vi "CANOpen_Main_Emergency.vi"(6 "EM GB NG conf":T3(array[cluster])=[{"Emergency"={"Enable"=TRUE}, "Heartbeat and Node Guarding"={"Mode"=enum."None", "Guard Time (ms)"=5, "Consumer Time (ms)"=5}}, {"Emergency"={"Enable"=TRUE}, "Heartbeat and Node Guarding"={"Mode"=enum."None", "Guard Time (ms)"=5, "Consumer Time (ms)"=5}}], 7 "Period":i64=10, 8 "error in (no error)":errorcluster, 9 "stop in":bool, 10 "Nodes":T4[](array[typedef])=[{"RPDOs"=[], "TPDOs"=[], "Node ID"=1, "SDOs"=[], "Dynamic SDOs"=[], "Node run state"=128, "Emergency"=FALSE, "HB NG"={"Mode"=enum."None", "Update Time"=5, "Static detect in None"=enum."HB"}, "Delay for opp. state (ms)"=1000.0, "Node init static SDO state"=128, "Stop and Reset on Shutdown"=FALSE}, {"RPDOs"=[], "TPDOs"=[], "Node ID"=2, "SDOs"=[], "Dynamic SDOs"=[], "Node run state"=128, "Emergency"=FALSE, "HB NG"={"Mode"=enum."None", "Update Time"=5, "Static detect in None"=enum."HB"}, "Delay for opp. state (ms)"=1000.0, "Node init static SDO state"=128, "Stop and Reset on Shutdown"=FALSE}] {"Node init static SDO state" items=["start remote node"=1, "enter pre-operational"=128]; "Node run state" items=["start remote node"=1, "stop remote node"=2, "enter pre-operational"=128, "reset node"=129, "reset communication"=130]; "RPDOs"."PDO Channel" items=["PDO 1", "PDO 2", "PDO 3", "PDO 4"]; "RPDOs"."Parameters"."Bit Offset" max=8 step=1; "RPDOs"."Parameters"."Byte Offset" max=8 step=1; "TPDOs"."PDO Channel" items=["PDO 1", "PDO 2", "PDO 3", "PDO 4"]; "TPDOs"."Parameters"."Bit Offset" max=8 step=1; "TPDOs"."Parameters"."Byte Offset" max=8 step=1}, 11 "interface object in":refnum<k20>) -> (0 "error out":errorcluster, 1 "Timestamp":timestamp, 2 "emergency message":T11 {"manufacturer specific error field" format="%.0x"; "error register" format="%.0x"; "error code" format="%.0x"}, 3 "interface object out":refnum<k20>, 5 "Is New?":bool)   [LabVIEW 2013, in "CANOpen Addon Custom Device.lvlib"]
uses:
  CANOpen Addon Custom Device.lvlib
  SubVIS/CANOpen_Node Message Settings.ctl
  Shared Code/CANOpen_PDO Settings.ctl
  Shared Code/CANOpen_PDO Parameter Settings.ctl
  Shared Code/CANOpen_PDO Data Type.ctl
  Shared Code/CANOpen_SDO Settings.ctl
  CanOpen_NMT_Config.ctl
  CanOpen_NMT_Static detect.ctl
  Shared Code/CANOpen_Emergency Settings.ctl
  Shared Code/CANOpen_Heartbeat and Node Guarding Settings.ctl
  Emergency VI states.ctl
  <vilib>/Platform/TimedLoop/XDataNode/timing_clust.ctl
  <vilib>/Platform/TimedLoop/XDataNode/nitl_modes.ctl
  <vilib>/Platform/TimedLoop/XDataNode/wakeup.ctl
  <vilib>/CANopenLib/CANOPEN.llb/CANopen Heartbeat Create.vi
  <vilib>/CANopenLib/CANOPEN.llb/CANopen Heartbeat Start.vi
  <vilib>/CANopenLib/CANOPEN.llb/CANopen Heartbeat State Read.vi
  <vilib>/CANopenLib/CANOPEN.llb/CANopen Heartbeat Close.vi
  <vilib>/CANopenLib/CANOPEN.llb/CANopen Emergency Create.vi
  <vilib>/CANopenLib/CANOPEN.llb/CANopen Emergency Start.vi
  <vilib>/CANopenLib/CANOPEN.llb/CANopen Emergency Read.vi
  <vilib>/CANopenLib/CANOPEN.llb/CANopen Emergency Close.vi
  <vilib>/CANopenLib/CANOPEN.llb/CANopen Node Guarding Create.vi
  <vilib>/CANopenLib/CANOPEN.llb/CANopen Node Guarding Start.vi
  <vilib>/CANopenLib/CANOPEN.llb/CANopen Node Guarding State Read.vi
  <vilib>/CANopenLib/CANOPEN.llb/CANopen Node Guarding Close.vi
  <vilib>/Platform/TimedLoop/XDataNode/XDataNode.xnode
  <vilib>/Platform/TimedLoop/XDataNode/XDNodeRunTimeDep.lvlib
panel:
  out "timestamp 2":timestamp
  out "state 2":u16(ring) items=["unknown"=1, "bootup"=0, "stopped"=4, "operational"=5, "pre-operational"=127, "connection lost"=128]
  out "error out 3":errorcluster
  out "state":u16(ring) items=["unknown"=1, "bootup"=0, "stopped"=4, "operational"=5, "pre-operational"=127, "connection lost"=128]
  out "timestamp":timestamp
  out "error out 2":errorcluster
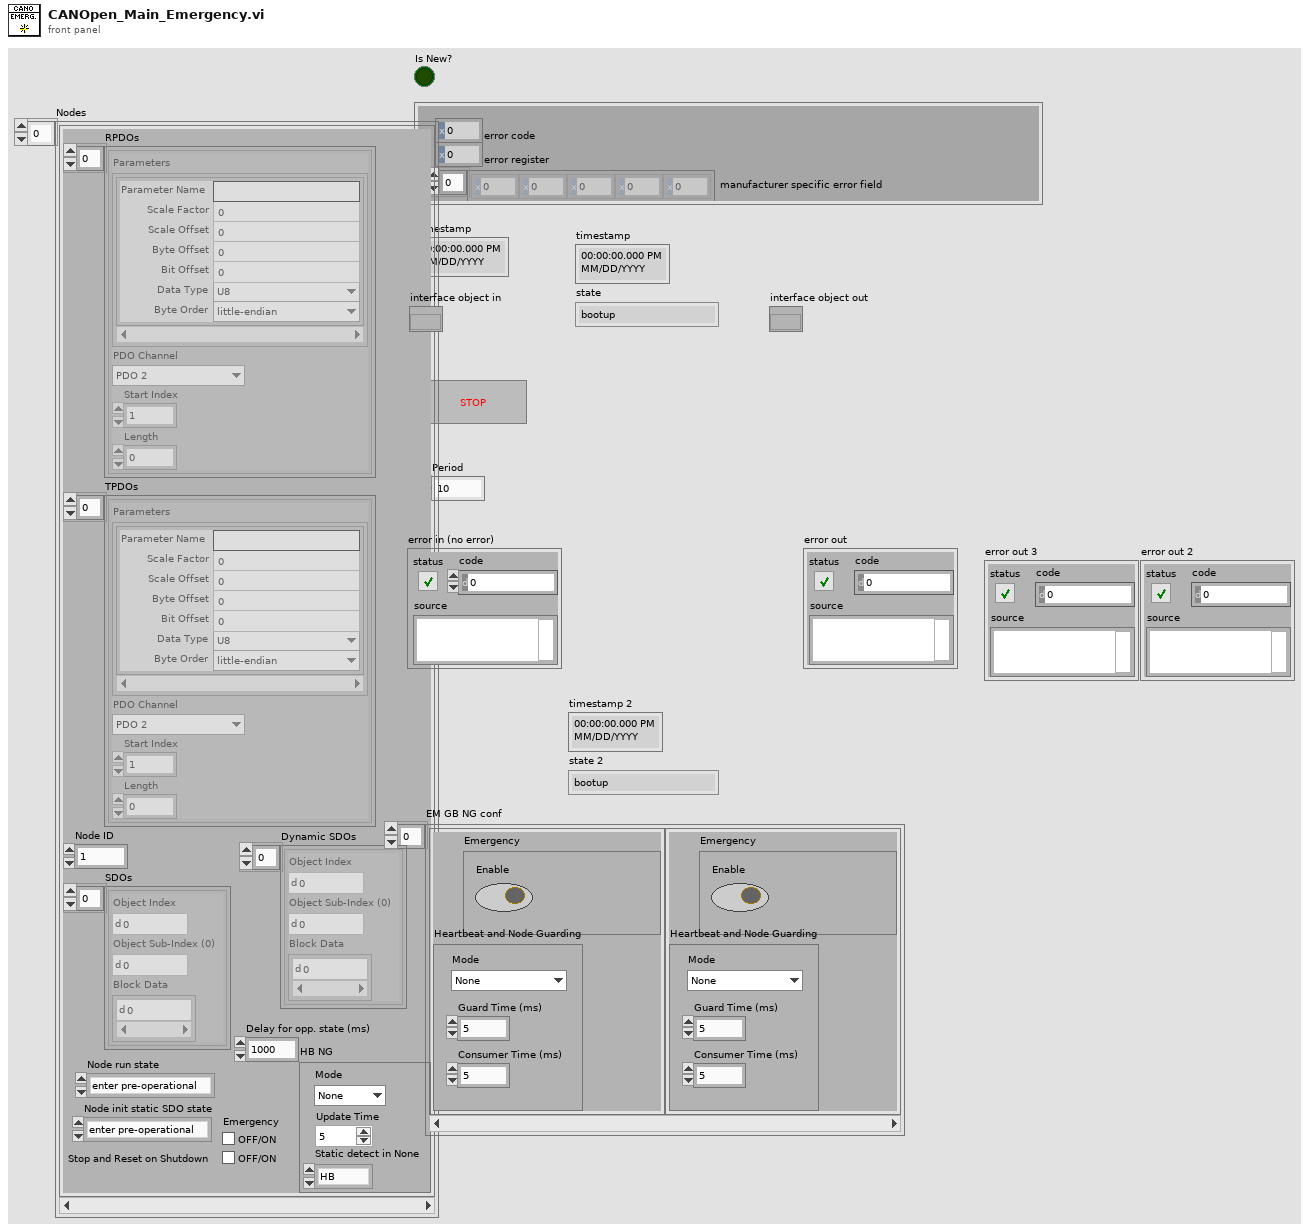
[diagram p1: front panel]
types:
  T1 = typedef "CANOpen Addon Custom Device.lvlib/CANOpen_Emergency Settings.ctl" = cluster{"Enable":bool}
  T2 = typedef "CANOpen Addon Custom Device.lvlib/CANOpen_Heartbeat and Node Guarding Settings.ctl" = cluster{"Mode":enum16{"None", "Hearbeat", "Node Guarding"}, "Guard Time (ms)":u16, "Consumer Time (ms)":u16}
  T3 = cluster{"Emergency":T1, "Heartbeat and Node Guarding":T2}[]
  T4 = typedef "CANOpen_Node Message Settings.ctl" = cluster{"RPDOs":T5[], "TPDOs":T5[], "Node ID":u8, "SDOs":T8[], "Dynamic SDOs":T8[], "Node run state":u16, "Emergency":bool, "HB NG":T9, "Delay for opp. state (ms)":dbl, "Node init static SDO state":u16, "Stop and Reset on Shutdown":bool}
  T5 = typedef "CANOpen Addon Custom Device.lvlib/CANOpen_PDO Settings.ctl" = cluster{"Parameters":T6[], "PDO Channel":u8, "Start Index":u32, "Length":u32}
  T6 = typedef "CANOpen Addon Custom Device.lvlib/CANOpen_PDO Parameter Settings.ctl" = cluster{"Parameter Name":string, "Scale Factor":dbl, "Scale Offset":dbl, "Byte Offset":u8, "Bit Offset":u8, "Data Type":T7, "Byte Order":enum16{"big-endian, network order", "little-endian"}}
  T7 = typedef "CANOpen Addon Custom Device.lvlib/CANOpen_PDO Data Type.ctl" = enum16{"U8", "U16", "U32", "I8", "I16", "I32", "Single", "Double", "Boolean"}
  T8 = typedef "CANOpen Addon Custom Device.lvlib/CANOpen_SDO Settings.ctl" = cluster{"Object Index":u16, "Object Sub-Index (0)":u8, "Block Data":u8[]}
  T9 = typedef "CANOpen Addon Custom Device.lvlib/CanOpen_NMT_Config.ctl" = cluster{"Mode":enum16{"None", "HB", "NG"}, "Update Time":u16, "Static detect in None":T10}
  T10 = typedef "CANOpen Addon Custom Device.lvlib/CanOpen_NMT_Static detect.ctl" = enum16{"None", "HB", "NG"}
  T11 = cluster{"error code":u16, "error register":u8, "manufacturer specific error field":u8[]}
  T12 = typedef "CANOpen Addon Custom Device.lvlib/Emergency VI states.ctl" = enum16{"Init", "Running ", "Shutdown"}
  T13 = typedef "XDNodeRunTimeDep.lvlib/timing_clust.ctl" = cluster{"Expected End [f-1]":u64, "Actual End [f-1]":u64, "Finished Late? [f-1]":bool, "Expected End [i-1]":u64, "Actual End [i-1]":u64, "Finished Late? [i-1]":bool, "Expected Start [i]":u64, "Actual Start [i]":u64, "Expected Start [f]":u64, "Actual Start [f]":u64, "Source Name":string, "Structure Name":string, "Period":i64, "Deadline":i64, "Offset":i64, "Start":i64, "Priority":i32, "Timeout":i32, "Mode":T14, "Wakeup Reason":T15, "Error":errorcluster, "Source Type":string, "Secondary Source Type":string, "Global End Time":u64, "Global Start Time":u64, "Frame Duration":u64, "Iteration Duration":u64, "Assigned CPU":i32, "I/O Scan Engine Mode":u32}
  T14 = typedef "XDNodeRunTimeDep.lvlib/nitl_modes.ctl" = enum32{"No Change", "Process missed periods, maintain original phase", "Discard missed periods, maintain original phase", "Process missed periods, ignore original phase", "Discard missed periods, ignore original phase"}
  T15 = typedef "XDNodeRunTimeDep.lvlib/wakeup.ctl" = enum32{"Normal", "Aborted", "Asynchronous wakeup", "Timing source error", "Timed loop error", "Timeout"}
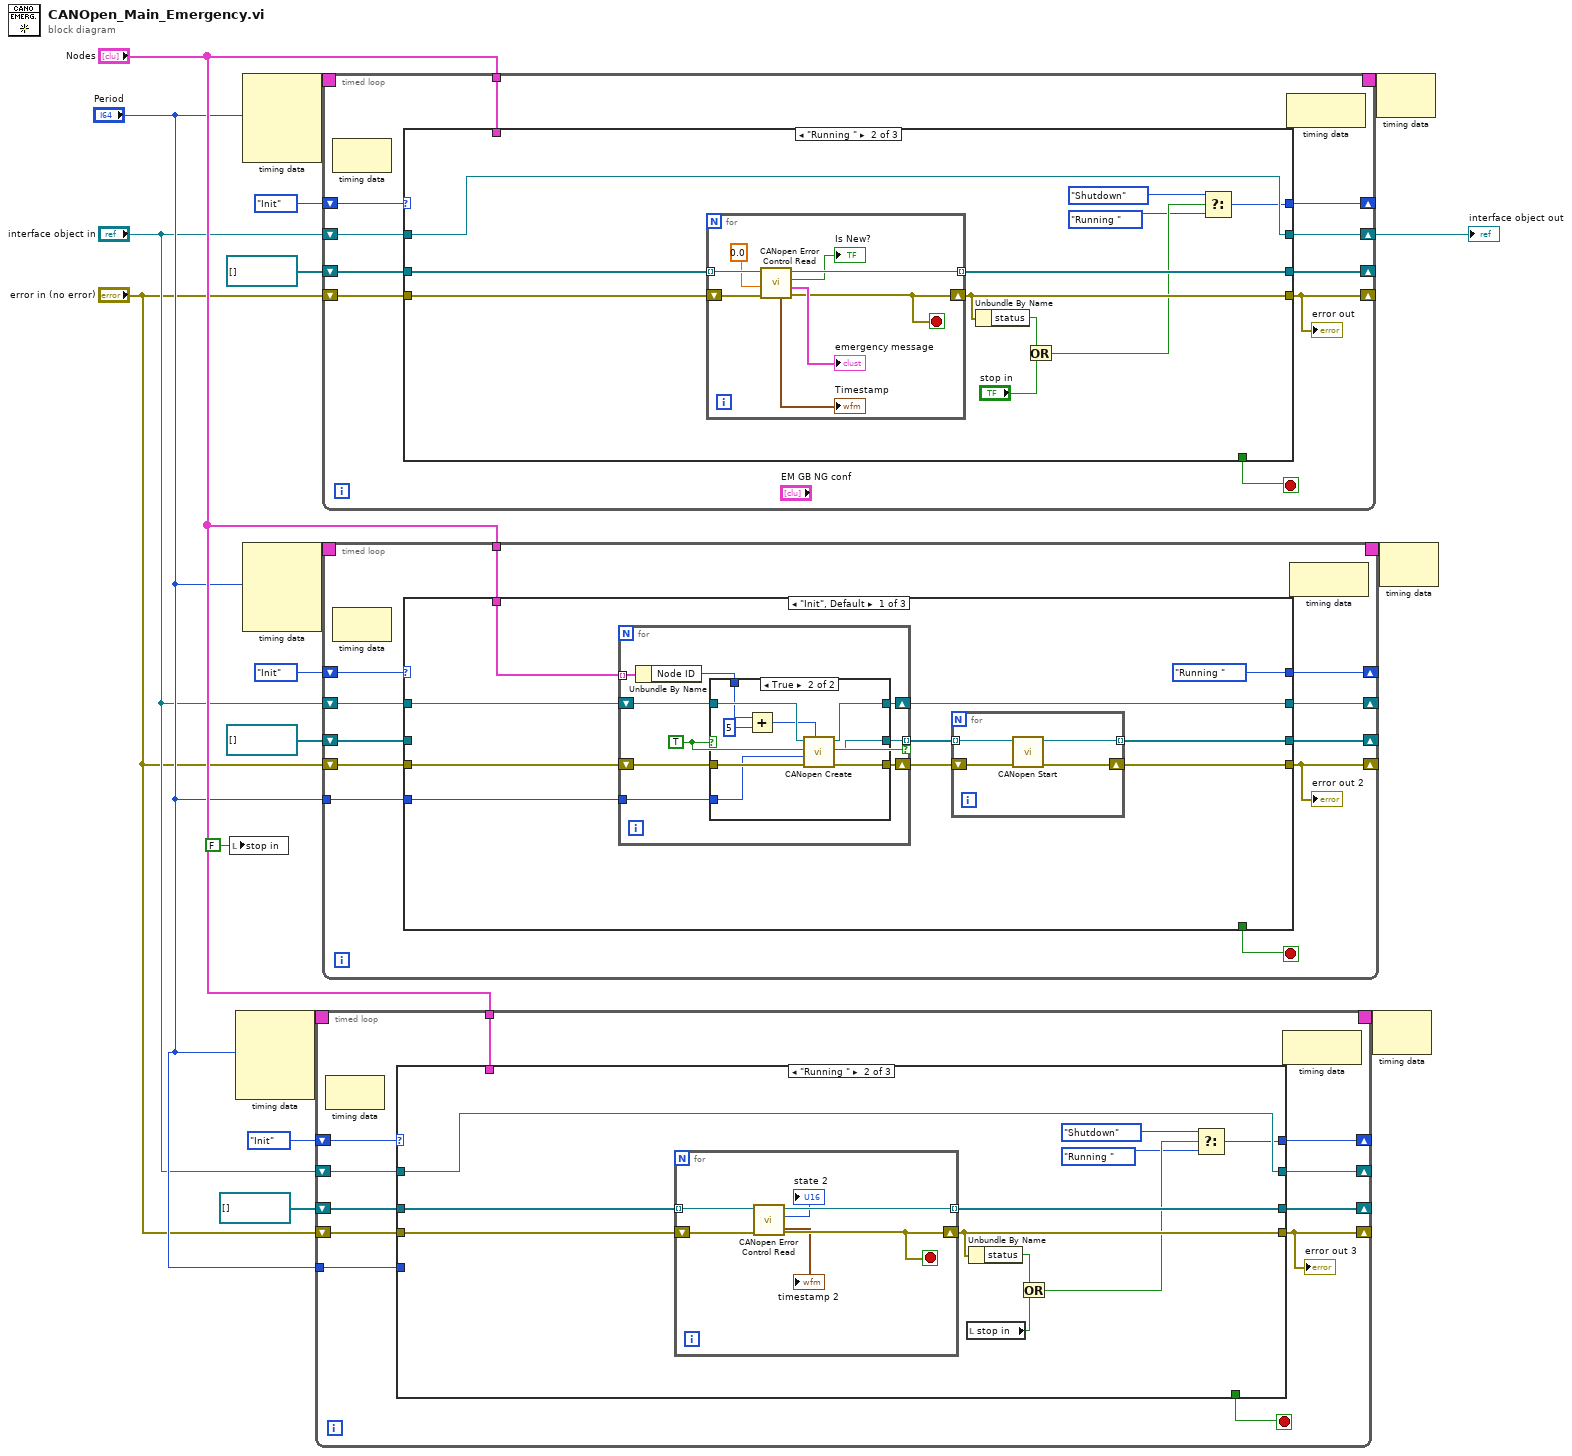
[diagram p0: block diagram]
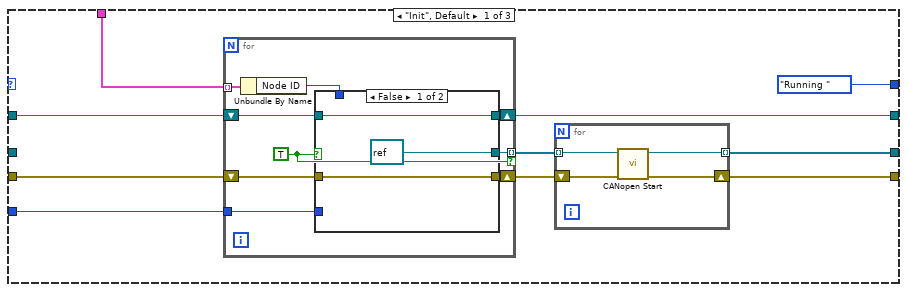
[diagram p2: hidden frame]
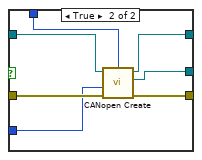
[diagram p3: hidden frame]
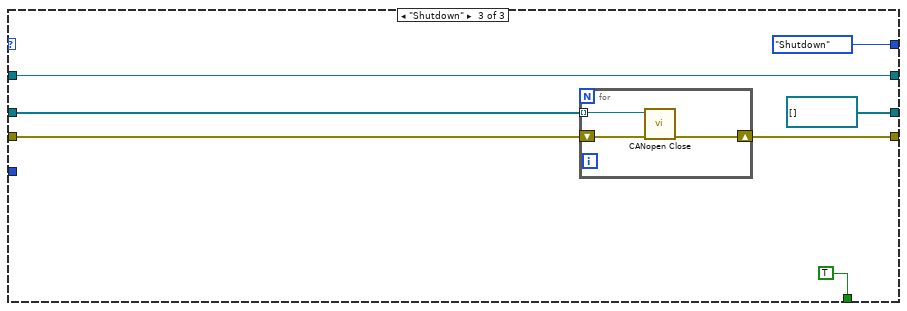
[diagram p4: hidden frame]
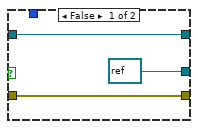
[diagram p5: hidden frame]
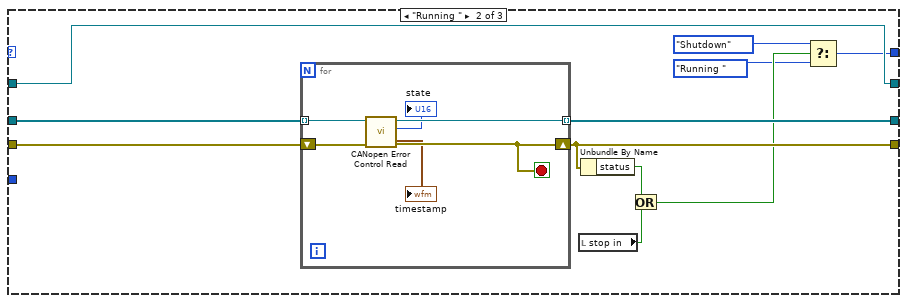
[diagram p6: hidden frame]
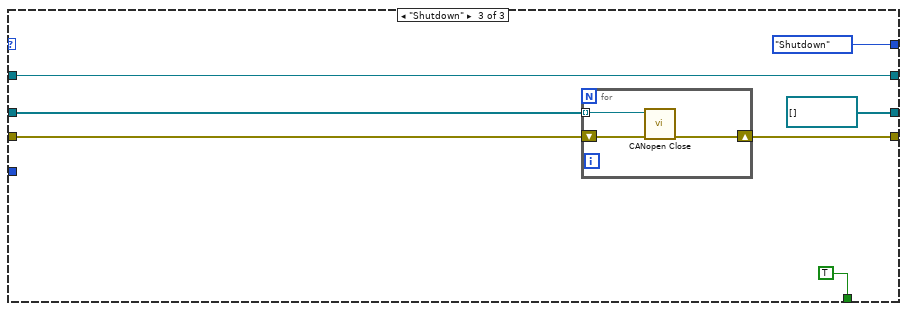
[diagram p7: hidden frame]
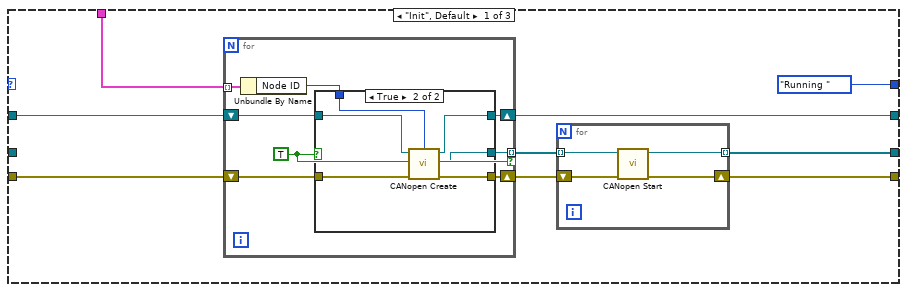
[diagram p8: hidden frame]
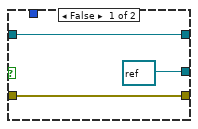
[diagram p9: hidden frame]
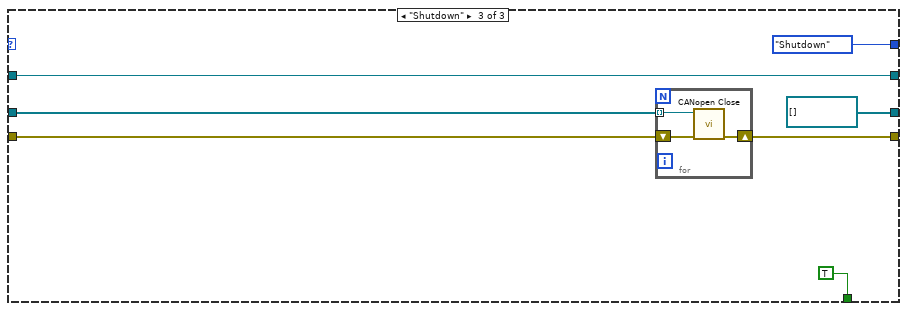
[diagram p10: hidden frame]
diagram:
  n1 = local write "stop in"(FALSE ("stop in")) -> ()
  n2 = node-c288("Period") -> (w8:T13)  [unwired: 3 in]
  n3 = node-c288("Period") -> (w16:T13)  [unwired: 3 in]
  n4 = node-c288("Period") -> (w13:T13)  [unwired: 3 in]
  n5 = timed-loop {
    shift-right: [w28] -> _
    shift-left: Emergency_VI_states."Init" -> [w29]
    shift-right: [w23] -> _
    shift-left: refnum<k20>[] [] -> [w25]
    shift-right: [w21] -> _
    shift-left: "error in (no error)" -> [w26]
    shift-right: [w24] -> _
    shift-left: "interface object in" -> [w22]
    timing: w8 -> [_]
    timing-out: [_] -> w7
    tunnel: "Nodes" -> [w20]
    tunnel: "Period" -> [w19]
    stop <- w27 stop-if-true
    n6 = node-c288() -> ()  [unwired: 1 in, 1 out]
    n7 = case shown="\"Running \"" w29 {
      tunnel: [Emergency_VI_states."Running " w68 Emergency_VI_states."Shutdown"] -> w28
      tunnel: [_ _ TRUE] -> w27
      tunnel: w26 -> [w33 w71 w85]
      tunnel: [w39 w70 w84] -> w21
      tunnel: w25 -> [_ w75 w86]
      tunnel: [w38 w73 w87] -> w24
      tunnel: [w37 w74 refnum<k20>[] []] -> w23
      tunnel: w22 -> [w35 w73 w87]
      tunnel: w20 -> [w34 _ _]
      tunnel: w19 -> [w32 _ _]
      frame "Init", Default {
        n8 = for {
          tunnel: w34 -> [w52] mode=indexing
          shift-right: [w54] -> w40
          shift-left: w33 -> [w51]
          shift-right: [w49] -> w38
          shift-left: w35 -> [w53]
          tunnel: [w48] -> w36 mode=indexing if=w47
          tunnel: w32 -> [w46]
          w47 = TRUE
          n9 = Unbundle By Name(w52) -> ("Node ID"=w50:u8)
          n10 = case shown="False" w47 {
            tunnel: [w57 w64] -> w54
            tunnel: [refnum<k20> refnum ("node guarding object out") w63] -> w48
            tunnel: w53 -> [w56 w62]
            tunnel: w51 -> [w57 w61]
            tunnel: w50 -> [_ w60]
            tunnel: [w56 w59] -> w49
            tunnel: w46 -> [_ w58]
            frame False {
            }
            frame True {
              n11 = call-poly <vilib>:"CANopen Create.vi"("node-ID"=w60, "error in (no error)"=w61, "guard time [ms]"=w58, "interface object in"=w62) -> ("error out"=w64:errorcluster, "node guarding object out"=w63:refnum<k20>, "interface object out"=w59:refnum<k20>)  [unwired: 5 in]
            }
          }
        }
        n12 = for {
          tunnel: w36 -> [w44] mode=indexing
          tunnel: [w42] -> w37 mode=indexing
          shift-right: [w43] -> w39
          shift-left: w40 -> [w45]
          n13 = call-poly <vilib>:"CANopen Start.vi"("error in (no error)"=w45, "node guarding object in"=w44) -> ("error out"=w43:errorcluster, "node guarding object out"=w42:refnum<k20>)  [unwired: 8 in]
        }
      }
      frame "Running " {
        n14 = for {
          tunnel: w75 -> [w81] mode=indexing
          tunnel: [w80] -> w74 mode=indexing
          shift-right: [w78] -> w70
          shift-left: w71 -> [w79]
          stop <- w78 stop-if-true
          n15 = call-poly <vilib>:"CANopen Error Control Read.vi"("error in (no error)"=w79, "node guarding object in"=w81) -> ("error out"=w78:errorcluster, "state"=→"state 2":u16, "node guarding object out"=w80:refnum<k20>, "timestamp"=→"timestamp 2":timestamp)  [unwired: 6 in]
        }
        n16 = local read "stop in"() -> (w65:bool)
        n17 = Unbundle By Name(w70) -> ("status"=w72:bool)
        n18 = Or(x=w72, y=w65) -> (x .or. y?=w69:bool)
        n19 = Select(t=Emergency_VI_states."Shutdown", s=w69, f=Emergency_VI_states."Running ") -> (s? t:f=w68:T12)
      }
      frame "Shutdown" {
        n20 = for {
          shift-right: [w90] -> w84
          shift-left: w85 -> [w91]
          tunnel: w86 -> [w89] mode=indexing
          n21 = call-poly <vilib>:"CANopen Close.vi"("error in (no error)"=w91, "node guarding object in"=w89) -> ("error out"=w90:errorcluster)  [unwired: 9 in]
        }
      }
    }
    "error out 3" <- w21
    n22 = node-c288() -> ()  [unwired: 1 in, 1 out]
  }
  n23 = timed-loop {
    shift-right: [w100] -> _
    shift-left: Emergency_VI_states."Init" -> [w101]
    shift-right: [w95] -> _
    shift-left: refnum<k20>[] [] -> [w97]
    shift-right: [w93] -> _
    shift-left: "error in (no error)" -> [w98]
    shift-right: [w96] -> w14
    shift-left: "interface object in" -> [w94]
    timing: w16 -> [_]
    timing-out: [_] -> w15
    tunnel: "Nodes" -> [w92]
    stop <- w99 stop-if-true
    n24 = node-c288() -> ()  [unwired: 1 in, 1 out]
    n25 = case shown="\"Running \"" w101 {
      tunnel: [Emergency_VI_states."Running " w136 Emergency_VI_states."Shutdown"] -> w100
      tunnel: [_ _ TRUE] -> w99
      tunnel: w98 -> [w104 w139 w156]
      tunnel: [w110 w138 w155] -> w93
      tunnel: w97 -> [_ w144 w157]
      tunnel: [w109 w142 w158] -> w96
      tunnel: [w108 w143 refnum<k20>[] []] -> w95
      tunnel: w94 -> [w106 w142 w158]
      tunnel: w92 -> [w105 _ _]
      frame "Init", Default {
        n26 = for {
          tunnel: w105 -> [w122] mode=indexing
          shift-right: [w124] -> w111
          shift-left: w104 -> [w121]
          shift-right: [w119] -> w109
          shift-left: w106 -> [w123]
          tunnel: [w118] -> w107 mode=indexing if=w117
          w117 = TRUE
          n27 = Unbundle By Name(w122) -> ("Node ID"=w120:u8)
          n28 = case shown="True" w117 {
            tunnel: [w127 w133] -> w124
            tunnel: [refnum<k20> refnum ("emergency object out") w132] -> w118
            tunnel: w123 -> [w126 w131]
            tunnel: w121 -> [w127 w130]
            tunnel: w120 -> [_ w129]
            tunnel: [w126 w128] -> w119
            frame False {
            }
            frame True {
              n29 = call-poly <vilib>:"CANopen Create.vi"("node-ID"=w129, "error in (no error)"=w130, "interface object in"=w131) -> ("error out"=w133:errorcluster, "emergency object out"=w132:refnum<k20>, "interface object out"=w128:refnum<k20>)  [unwired: 6 in]
            }
          }
        }
        n30 = for {
          tunnel: w107 -> [w115] mode=indexing
          tunnel: [w113] -> w108 mode=indexing
          shift-right: [w114] -> w110
          shift-left: w111 -> [w116]
          n31 = call-poly <vilib>:"CANopen Start.vi"("error in (no error)"=w116, "emergency object in"=w115) -> ("error out"=w114:errorcluster, "emergency object out"=w113:refnum<k20>)  [unwired: 8 in]
        }
      }
      frame "Running " {
        n32 = for {
          tunnel: w144 -> [w151] mode=indexing
          tunnel: [w150] -> w143 mode=indexing
          shift-right: [w145] -> w138
          shift-left: w139 -> [w146]
          stop <- w145 stop-if-true
          n33 = call-poly <vilib>:"CANopen Error Control Read.vi"("error in (no error)"=w146, "timeout (0s)"=0.0 ("timeout(0)"), "emergency object in"=w151) -> ("error out"=w145:errorcluster, "emergency message"=→"emergency message":T11, "new message?"=→"Is New?":bool, "emergency object out"=w150:refnum<k20>, "timestamp"=→"Timestamp":timestamp)  [unwired: 4 in]
        }
        n34 = Unbundle By Name(w138) -> ("status"=w140:bool)
        n35 = Or(x=w140, y="stop in") -> (x .or. y?=w137:bool)
        n36 = Select(t=Emergency_VI_states."Shutdown", s=w137, f=Emergency_VI_states."Running ") -> (s? t:f=w136:T12)
      }
      frame "Shutdown" {
        n37 = for {
          shift-right: [w162] -> w155
          shift-left: w156 -> [w161]
          tunnel: w157 -> [w160] mode=indexing
          n38 = call-poly <vilib>:"CANopen Close.vi"("error in (no error)"=w161, "emergency object in"=w160) -> ("error out"=w162:errorcluster)  [unwired: 9 in]
        }
      }
    }
    "error out" <- w93
    n39 = node-c288() -> ()  [unwired: 1 in, 1 out]
  }
  "interface object out" <- w14
  n40 = timed-loop {
    shift-right: [w172] -> _
    shift-left: Emergency_VI_states."Init" -> [w173]
    shift-right: [w167] -> _
    shift-left: refnum<k20>[] [] -> [w169]
    shift-right: [w165] -> _
    shift-left: "error in (no error)" -> [w170]
    shift-right: [w168] -> _
    shift-left: "interface object in" -> [w166]
    timing: w13 -> [_]
    timing-out: [_] -> w12
    tunnel: "Nodes" -> [w164]
    tunnel: "Period" -> [w163]
    stop <- w171 stop-if-true
    n41 = node-c288() -> ()  [unwired: 1 in, 1 out]
    n42 = case shown="\"Init\", Default" w173 {
      tunnel: [Emergency_VI_states."Running " w214 Emergency_VI_states."Shutdown"] -> w172
      tunnel: [_ _ TRUE] -> w171
      tunnel: w170 -> [w177 w217 w231]
      tunnel: [w183 w216 w230] -> w165
      tunnel: w169 -> [_ w221 w232]
      tunnel: [w182 w219 w233] -> w168
      tunnel: [w181 w220 refnum<k20>[] []] -> w167
      tunnel: w166 -> [w179 w219 w233]
      tunnel: w164 -> [w178 _ _]
      tunnel: w163 -> [w176 _ _]
      frame "Init", Default {
        n43 = for {
          tunnel: w178 -> [w196] mode=indexing
          shift-right: [w198] -> w184
          shift-left: w177 -> [w195]
          shift-right: [w193] -> w182
          shift-left: w179 -> [w197]
          tunnel: [w192] -> w180 mode=indexing if=w191
          tunnel: w176 -> [w190]
          w191 = TRUE
          n44 = Unbundle By Name(w196) -> ("Node ID"=w194:u8)
          n45 = case shown="True" w191 {
            tunnel: [w201 w210] -> w198
            tunnel: [refnum<k20> refnum ("heartbeat object out") w209] -> w192
            tunnel: w197 -> [w200 w208]
            tunnel: w195 -> [w201 w207]
            tunnel: w194 -> [_ w204]
            tunnel: [w200 w206] -> w193
            tunnel: w190 -> [_ w205]
            frame False {
            }
            frame True {
              n46 = Add(x=w204, y=u8 5) -> (x+y=w202:u8)
              n47 = call-poly <vilib>:"CANopen Create.vi"("node-ID"=w202, "error in (no error)"=w207, "consumer time [ms]"=w205, "interface object in"=w208) -> ("error out"=w210:errorcluster, "heartbeat object out"=w209:refnum<k20>, "interface object out"=w206:refnum<k20>)  [unwired: 5 in]
            }
          }
        }
        n48 = for {
          tunnel: w180 -> [w188] mode=indexing
          tunnel: [w186] -> w181 mode=indexing
          shift-right: [w187] -> w183
          shift-left: w184 -> [w189]
          n49 = call-poly <vilib>:"CANopen Start.vi"("error in (no error)"=w189, "heartbeat object in"=w188) -> ("error out"=w187:errorcluster, "heartbeat object out"=w186:refnum<k20>)  [unwired: 8 in]
        }
      }
      frame "Running " {
        n50 = for {
          tunnel: w221 -> [w227] mode=indexing
          tunnel: [w226] -> w220 mode=indexing
          shift-right: [w224] -> w216
          shift-left: w217 -> [w225]
          stop <- w224 stop-if-true
          n51 = call-poly <vilib>:"CANopen Error Control Read.vi"("error in (no error)"=w225, "heartbeat object in"=w227) -> ("error out"=w224:errorcluster, "state"=→"state":u16, "heartbeat object out"=w226:refnum<k20>, "timestamp"=→"timestamp":timestamp)  [unwired: 6 in]
        }
        n52 = local read "stop in"() -> (w211:bool)
        n53 = Unbundle By Name(w216) -> ("status"=w218:bool)
        n54 = Or(x=w218, y=w211) -> (x .or. y?=w215:bool)
        n55 = Select(t=Emergency_VI_states."Shutdown", s=w215, f=Emergency_VI_states."Running ") -> (s? t:f=w214:T12)
      }
      frame "Shutdown" {
        n56 = for {
          shift-right: [w236] -> w230
          shift-left: w231 -> [w237]
          tunnel: w232 -> [w235] mode=indexing
          n57 = call-poly <vilib>:"CANopen Close.vi"("error in (no error)"=w237, "heartbeat object in"=w235) -> ("error out"=w236:errorcluster)  [unwired: 9 in]
        }
      }
    }
    "error out 2" <- w165
    n58 = node-c288() -> ()  [unwired: 1 in, 1 out]
  }
  n59 = node-c288(w7) -> ()  [unwired: 1 out]
  n60 = node-c288(w15) -> ()  [unwired: 1 out]
  n61 = node-c288(w12) -> ()  [unwired: 1 out]
